vi "GetDataEventCreatorName.vi"(8 "error in (no error)":errorcluster) -> (0 "error out":errorcluster, 1 "found":bool, 2 "data event creator":string)   [LabVIEW 2017, in "GlobalConfiguration.lvlib"]
uses:
  <vilib>/addons/InsightCM/Utilities/GlobalConfiguration/GlobalConfiguration.lvlib
  <vilib>/addons/PointValueMap/subVIs/Point_Read_string.vi
  <vilib>/addons/PointValueMap/PointValueMap.lvlib
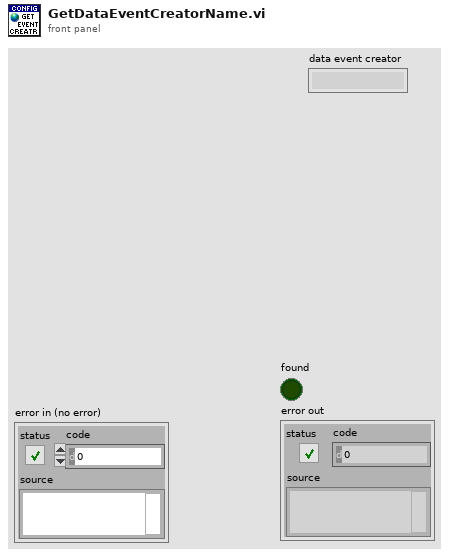
[diagram p1: front panel]
types:
  T1 = typedef "PointValueMap.lvlib/PointMap.ctl" = refnum<data-value>
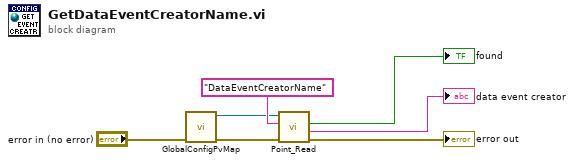
[diagram p0: block diagram]
diagram:
  n1 = call <vilib>:"GlobalConfigPvMap.vi"("error in (no error)"="error in (no error)") -> ("error out"=w4:errorcluster, "global configuration map"=w5:T1)  [unwired: 9 in]
  n2 = call-poly <vilib>:"Point_Read.vi"("Error In"=w4, "Tag"="DataEventCreatorName" ("Name"), "Map"=w5) -> ("Error Out"=→"error out":errorcluster, "Value"=→"data event creator":string, "Found?"=→"found":bool)  [unwired: 3 in, 3 out]
